vi "Topo & GridSpectr_DriftCorrection_v5 - Cloud.vi"(6 "Internal use":string, 7 "Grid param":T2 {"height (m)" format="%#_6p"; "width (m)" format="%#_6p"; "center Y (m)" format="%#_6p"; "center X (m)" format="%#_6p"}, 8 "Error in (no error)":errorcluster, 9 "Points Y/Index Y":i32, 10 "Points X/Index X":i32, 11 "Method":enum16{"init", "run", "end"}(ring)=enum."end") -> (0 "Error out":errorcluster)   [LabVIEW 2014]
doc: "Example of a measurement VI to be used in the \"Experiments on a Grid\" tool as external VI.\n\nThis example measure the topography and spectroscopy data. The spectroscopy measurements are taken on a subgrid. The data are saved to a sxm and a binary file.\n\n- Nanonis Programming Interface -"
uses:
  <userlib>/Nanonis Prog Interface V5/Nanonis Prog Interface.lvlib
panel:
  in  "Drift Correction":bool
  in  "Set Session":bool
  in  "STS current step":dbl format="%#_6p"
  in  "tip Speed (m/s)":sgl=1e-08 format="%.2p"
  in  "Drift Correction 2":T1
  out "X drift":i32
  out "Y drift":i32
  out "Queue Steps":i32=40
  in  "StepsBack":i32=40
  in  "Channel index (0-23)":u8=14
  in  "File name":string="_3_mol_Chain_single_mol_KONDO"
  in  "STS Current":dbl=2e-10 format="%#_6p"
  in  "Imaging Current":dbl=8e-11 format="%#_6p"
  in  "zdrift \nDuration (s)":dbl
  in  "Correct z drift":bool
  out "Status":string="init"
  in  "Drift correction Pixels":i32=256 caption="Pixels for drift correction"
  out "Y Offset":dbl
  out "X Offset":dbl
  out "Points taken":dbl
  in  "Drift Correction every":i32=10
  in  "Y subgrid spacing":u16=1
  in  "X subgrid spacing":u16=1
  # "drift corr. broken"
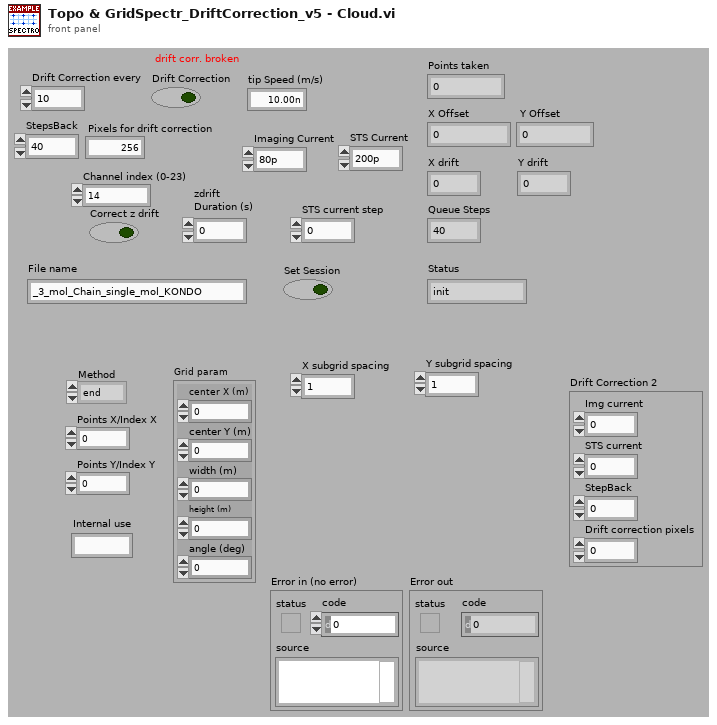
[diagram p1: front panel]
types:
  T1 = cluster{"Img current":dbl, "STS current":dbl, "StepBack":dbl, "Drift correction pixels":dbl}
  T2 = cluster{"center X (m)":sgl, "center Y (m)":sgl, "width (m)":sgl, "height (m)":sgl, "angle (deg)":sgl}
  T3 = enum16{"Header", "TOPO", "STS", "GRID", "GRIDCloud"}
  T4 = cluster{"center X":sgl, "center Y":sgl, "angle":sgl, "width":sgl, "height":sgl, "# pixels":i32, "# lines":i32}
  T5 = cluster{"Name":string, "Calibration":sgl, "Offset":sgl, "Channel index":i32}[]
  T6 = cluster{"up/down":bool, "time/line":sgl, "start time":timestamp, "end time":timestamp}
  T7 = cluster{"Z averaging time (s)":sgl, "Z offset (m)":sgl, "Initial settling time (s)":sgl}
  T8 = cluster{"Max. slew rate (V/s)":sgl, "Settling time (s)":sgl, "Integration time (s)":sgl}
  T9 = cluster{"End settling time (s)":sgl, "Z control time (s)":sgl}
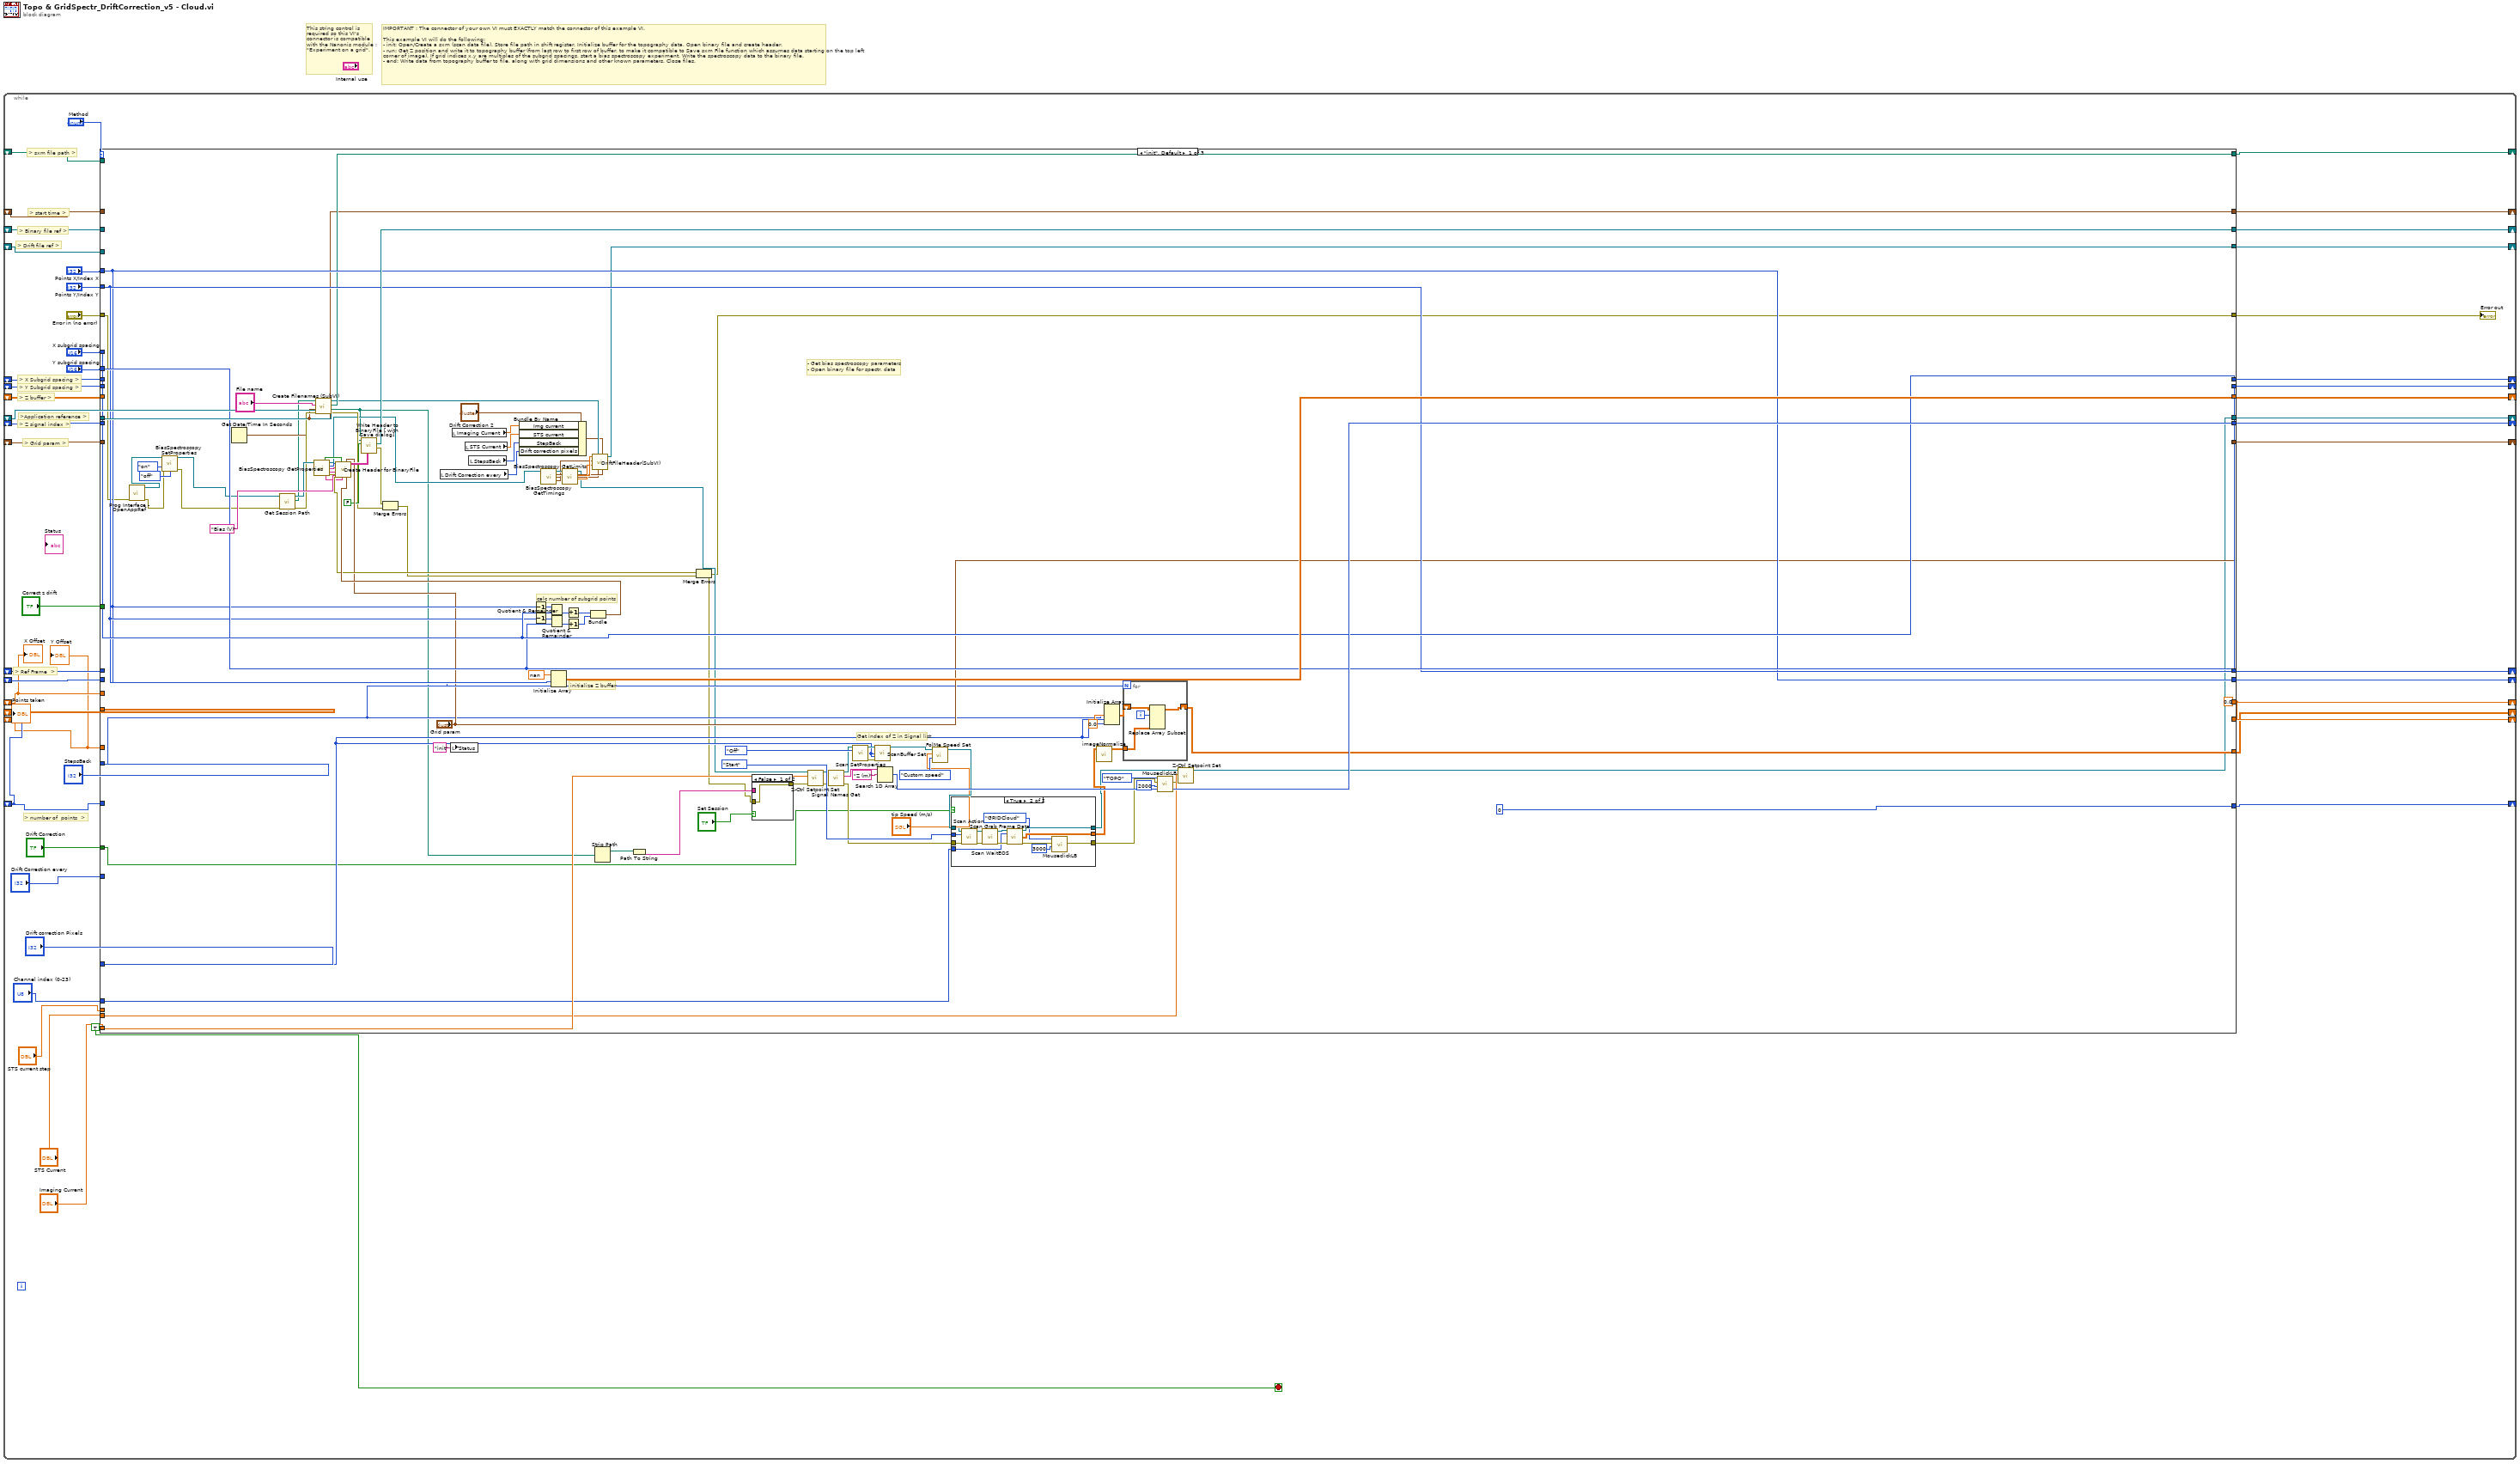
[diagram p0: block diagram]
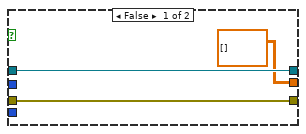
[diagram p2: hidden frame]
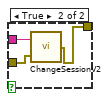
[diagram p3: hidden frame]
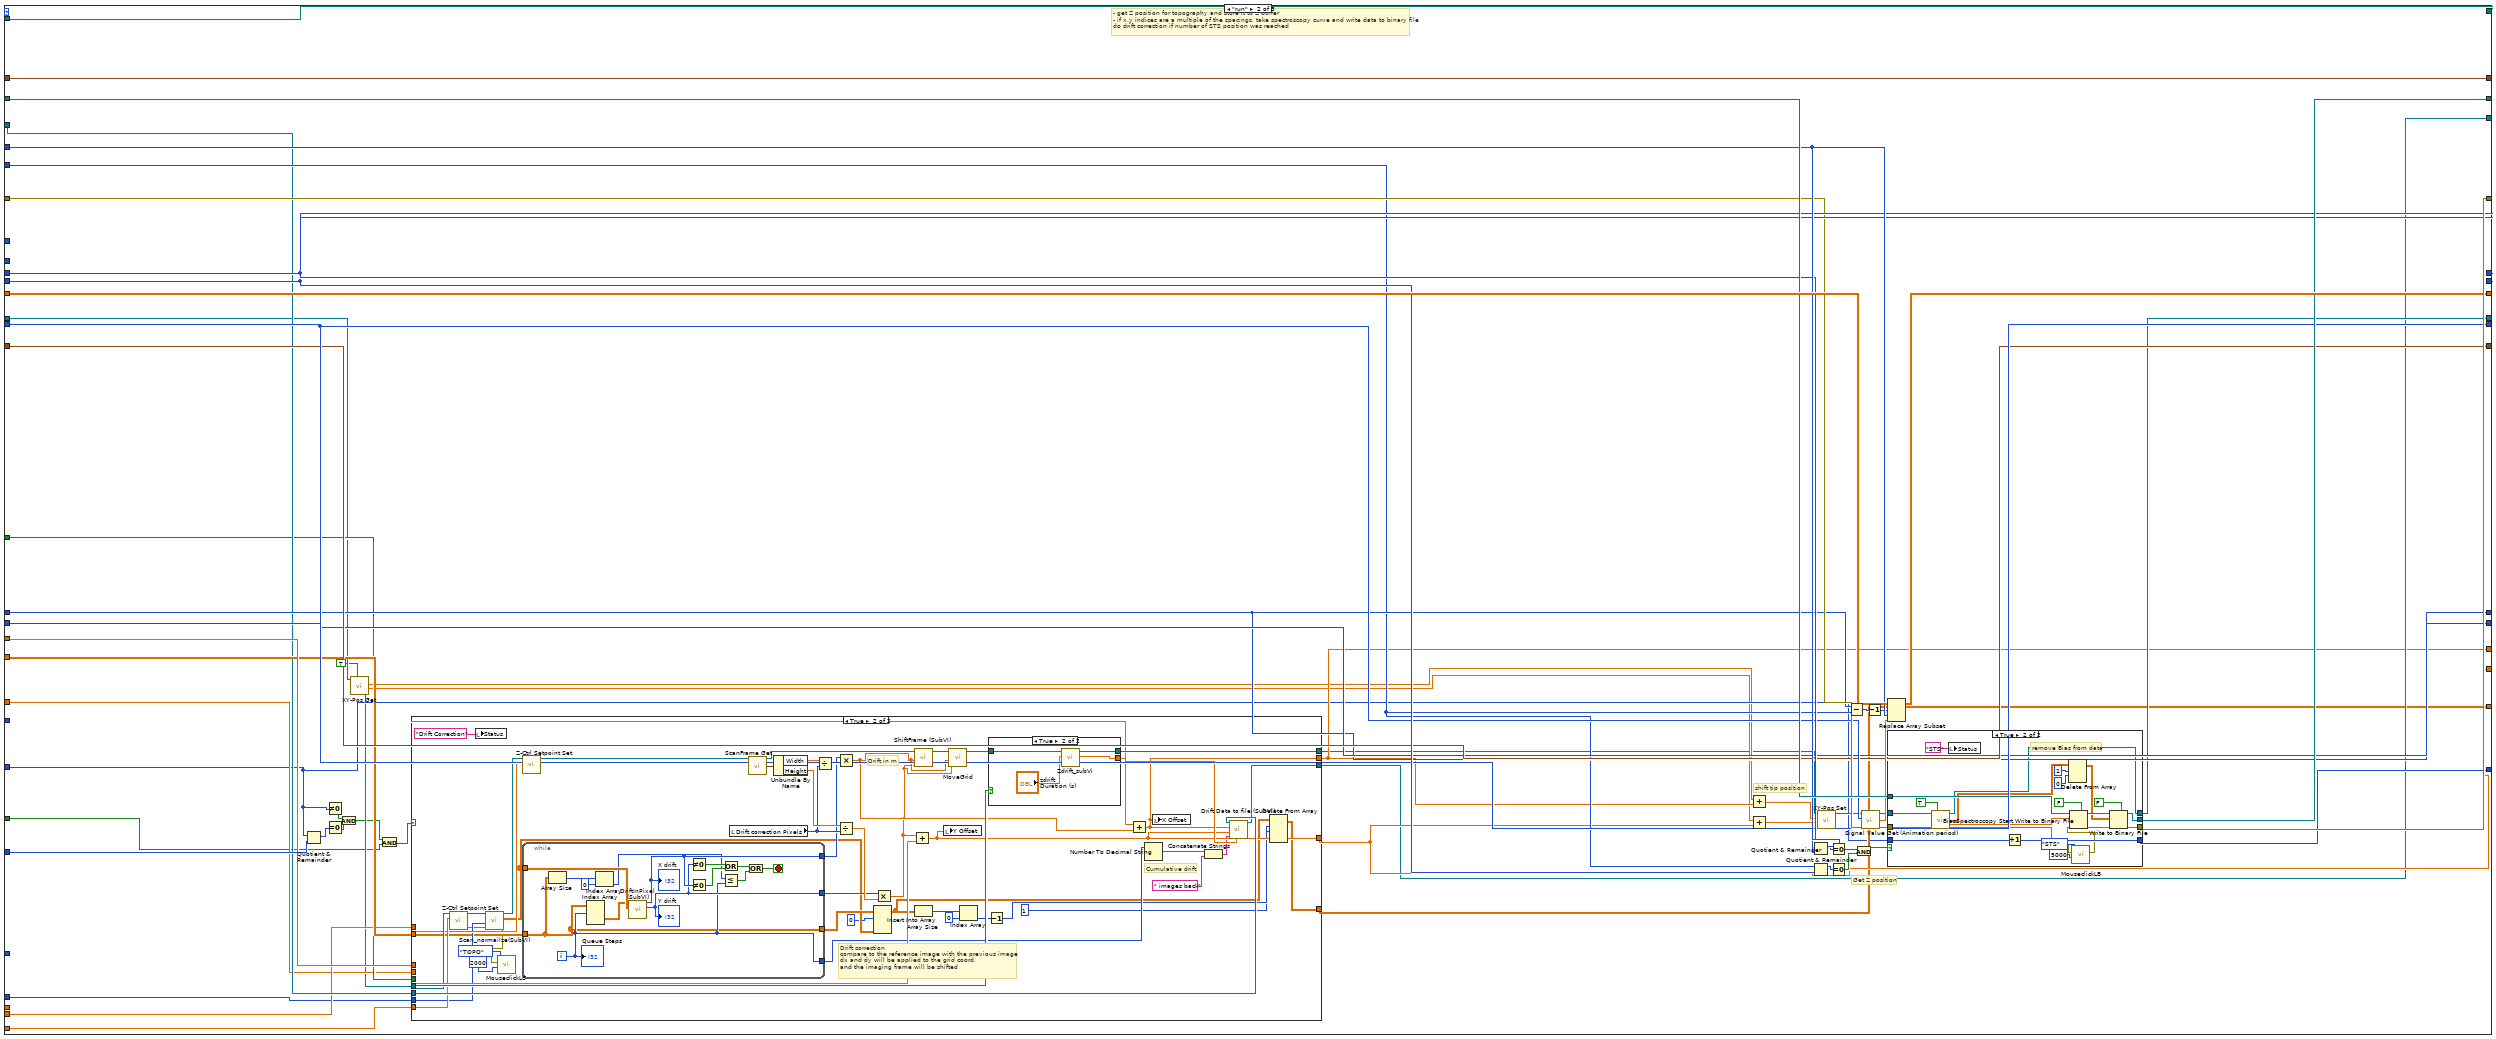
[diagram p4: hidden frame]
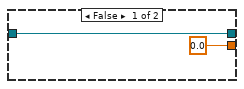
[diagram p6: hidden frame]
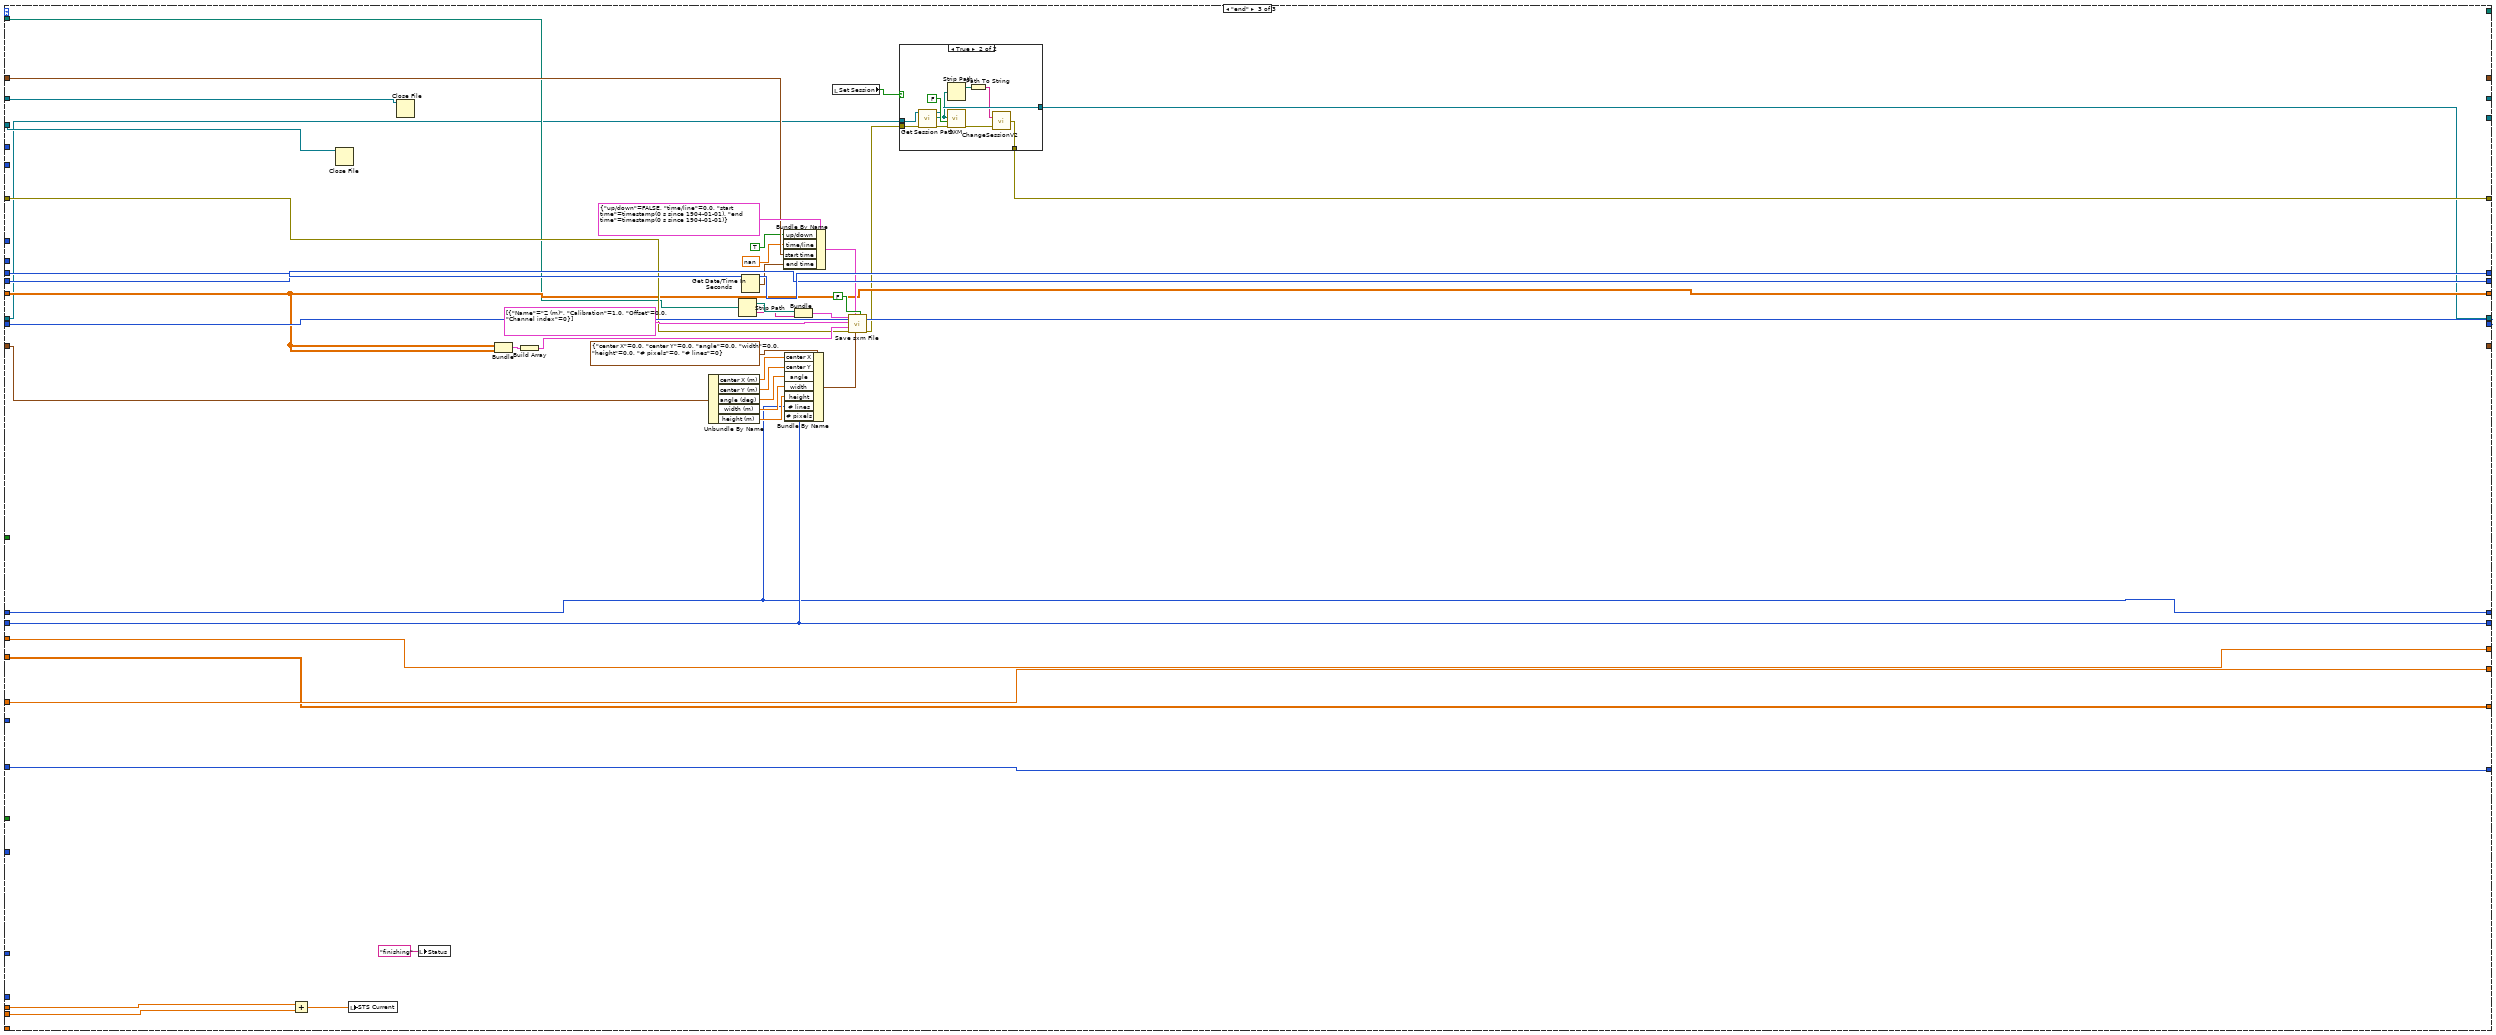
[diagram p8: hidden frame]
diagram:
  # "This string control is required so this VI's connector is compatible with the Nanonis module : \"Experiment on a grid\"."
  # "IMPORTANT : The connector of your own VI must EXACTLY match the connector of this example VI.\n\nThis example VI will do the following:\n- init: Open/Create a sxm (scan data file). Store file path in shift register. Initialize buffer for the topography data. Open binary file and create header.\n- run: Get Z position and write it to topography buffer (from last row to first row of buffer, to make it compatible to Save sxm File function which assumes data starting on the top left corner of image). If grid indices x,y are multiples of the subgrid spacings, start a bias spectroscopy experiment. Write the spectroscopy data to the binary file.\n- end: Write data from topography buffer to file, along with grid dimensions and other known parameters. Close files."
  n1 = while {
    shift-right: [w24] -> _
    shift-left: _ -> [w47]
    shift-right: [w42] -> _
    shift-left: _ -> [w41]
    shift-right: [w39] -> _
    shift-left: _ -> [w40]
    shift-right: [w38] -> _
    shift-left: _ -> [w37]
    shift-right: [w31] -> _
    shift-left: _ -> [w33]
    shift-right: [w32] -> _
    shift-left: _ -> [w34]
    shift-right: [w30] -> _
    shift-left: _ -> [w29]
    shift-right: [w28] -> _
    shift-left: _ -> [w27]
    shift-right: [w26] -> _
    shift-left: _ -> [w25]
    shift-right: [w23] -> _
    shift-left: _ -> [w22]
    shift-right: [w21] -> _
    shift-left: _ -> [w20]
    shift-right: [w19] -> _
    shift-left: _ -> [w12]
    shift-right: [w18] -> _
    shift-left: _ -> [w11]
    shift-right: [w17] -> _
    shift-left: _ -> [w14]
    shift-right: [w16] -> _
    shift-left: _ -> [w13]
    shift-right: [w9] -> _
    shift-left: _ -> [w8]
    stop <- TRUE stop-if-true
    # "> Drift file ref >"
    # "> number of  points  >"
    # "> Ref Frame  >"
    # "> Grid param >"
    # "> start time >"
    # ">Application reference >"
    # "> Y Subgrid spacing >"
    # "> X Subgrid spacing >"
    # "> Z signal index >"
    # "> Binary file ref >"
    # "> Z buffer >"
    # "> sxm file path >"
    n2 = case shown="\"init\", Default" "Method" {
      tunnel: [w102 w228 _] -> w24
      tunnel: w47 -> [_ w228 w336]
      tunnel: "Error in (no error)" -> [w63 w214 w359]
      tunnel: [w57 w227 w333] -> w45
      tunnel: "Points X/Index X" -> [w122 w222 _]
      tunnel: "Points Y/Index Y" -> [w123 w206 _]
      tunnel: [w146 w225 w348] -> w42
      tunnel: w41 -> [_ w226 w348]
      tunnel: w40 -> [_ w224 w337]
      tunnel: [w138 w223 _] -> w39
      tunnel: [w136 w212 w373] -> w38
      tunnel: w37 -> [_ w212 w373]
      tunnel: "X subgrid spacing" -> [w135 _ _]
      tunnel: "Y subgrid spacing" -> [w134 _ _]
      tunnel: w34 -> [_ w216 w372]
      tunnel: w33 -> [_ w215 w371]
      tunnel: [w135 w216 w372] -> w32
      tunnel: [w134 w215 w371] -> w31
      tunnel: [w75 w198 w331] -> w30
      tunnel: w29 -> [_ w180 w332]
      tunnel: ["Grid param" w209 _] -> w28
      tunnel: w27 -> [_ w209 w358]
      tunnel: [w101 w210 _] -> w26
      tunnel: w25 -> [_ w210 w366]
      tunnel: [w123 w207 w349] -> w23
      tunnel: w22 -> [_ w207 w349]
      tunnel: [w122 w208 w350] -> w21
      tunnel: w20 -> [_ w208 w350]
      tunnel: [w117 w188 w347] -> w19
      tunnel: [w117 w193 w345] -> w18
      tunnel: [w96 w185 w341] -> w17
      tunnel: [0 w203 w346] -> w16
      tunnel: w13 -> [_ w182 w346]
      tunnel: "Drift Correction every" -> [_ w201 _]
      tunnel: w14 -> [_ w192 w341]
      tunnel: w12 -> [_ w199 w347]
      tunnel: w11 -> [_ w183 w345]
      tunnel: "Drift correction Pixels" -> [w95 _ _]
      tunnel: [w91 w190 _] -> w9
      tunnel: w8 -> [_ w191 w342]
      tunnel: "Correct z drift" -> [_ w189 _]
      tunnel: "Imaging Current" -> [w108 w187 _]
      tunnel: "STS Current" -> [w105 w186 w338]
      tunnel: "Channel index (0-23)" -> [w99 w184 _]
      tunnel: "StepsBack" -> [w94 _ _]
      tunnel: "STS current step" -> [_ _ w340]
      tunnel: "Drift Correction" -> [w52 w172 _]
      frame "init", Default {
        w117 = 0.0
        # "- Get bias spectroscopy parameters\n- Open binary file for spectr. data"
        # "initialize Z buffer"
        # "calc number of subgrid points"
        # "Get index of Z in Signal list"
        n3 = call <userlib>:"Prog Interface - OpenAppRef.vi"("Error in (no error)"=w63) -> ("Error out"=w62:errorcluster, "Application reference"=w65:refnum<vi>)  [unwired: 5 in]
        n4 = call <userlib>:"BiasSpectroscopy SetProperties.vi"("Application ref in"=w65, "Autosave (no change)"=enum16{"no change", "on", "off"}."on", "Error in (no error)"=w62, "Save dialog"=enum16{"no change", "on", "off"}."off") -> ("Application ref out"=w64:refnum<vi>, "Error out"=w61:errorcluster)  [unwired: 10 in]
        n5 = Get Date/Time In Seconds() -> (seconds since 1Jan1904=w101:timestamp)
        n6 = call <userlib>:"Get Session Path.vi"("error in (no error)"=w61, "Application ref in"=w64) -> ("error out"=w103:errorcluster, "Session path"=w68:path, "Application ref out"=w104:refnum<vi>)  [unwired: 7 in]
        n7 = call <userlib>:"BiasSpectroscopy GetProperties.vi"("Application ref in"=w104) -> ("Backward sweep"=w142:bool, "Application ref out"=w74:refnum<vi>, "Number of points"=w125:i32, "Channels"=w124:string[], "Parameters"=w140:string[], "Fixed parameters"=w127:string[], "Error out"=w139:errorcluster)  [unwired: 6 in, 2 out]
        n8 = call "Create Filenames (SubVI).vi"("error in (no error)"=w103, "seconds since 1Jan1904"=w101, "File name"="File name", "Session path"=w68) -> ("error out"=w76:errorcluster, "binFilePath"=w58:path, "topoFilePath"=w102:path, "Drift File out"=w92:refnum<file>)  [unwired: 4 in]
        n9 = local read "Drift Correction every"() -> (w86:i32)
        n10 = local write "Status"("init" ("Status")) -> ()
        n11 = local read "Imaging Current"() -> (w88:dbl)
        n12 = local read "STS Current"() -> (w87:dbl)
        n13 = local read "StepsBack"() -> (w85:i32)
        n14 = Bundle By Name(cluster="Drift Correction 2", "Img current"=w88, "STS current"=w87, "StepBack"=w85, "Drift correction pixels"=w86) -> (w89:T1)
        n15 = Decrement(x=w122) -> (x-1=w133:i32)
        n16 = Decrement(x=w123) -> (x-1=w132:i32)
        n17 = call <userlib>:"BiasSpectroscopy GetTimings.vi"("Application ref in"=w74) -> ("Application ref out"=w84:refnum<vi>, "Initialization"=w81:T7, "Sweep Timing"=w79:T8, "End of Sweep"=w80:T9)  [unwired: 10 in, 1 out]
        n18 = Quotient & Remainder(x=w133, y=w135) -> (floor(x/y)=w131:i32)  [unwired: 1 out]
        n19 = Quotient & Remainder(x=w132, y=w134) -> (floor(x/y)=w130:i32)  [unwired: 1 out]
        n20 = Initialize Array(sgl nan ("element"), w123, w122) -> (w146:sgl[][])
        n21 = call <userlib>:"BiasSpectroscopy GetLimits.vi"("Application ref in"=w84) -> ("End value (V)"=w82:sgl, "Start value (V)"=w83:sgl, "Application ref out"=w73:refnum<vi>)  [unwired: 5 in, 1 out]
        n22 = Increment(x=w131) -> (x+1=w129:i32)
        n23 = Increment(x=w130) -> (x+1=w128:i32)
        n24 = Bundle(w129, w128) -> (w141:cluster{i32, i32})  [unwired: 1 in]
        n25 = call <userlib>:"Create Header for BinaryFile.vi"("Grid points"=w141, "Grid param"="Grid param", "Fixed parameters"=w127, "Backward sweep"=w142, "Sweep signal"="Bias (V)" ("Sweep Signal"), "Parameters"=w140, "Channels"=w124, "Points per sweep"=w125) -> ("Header (fixed attributes)"=w144:string[][])  [unwired: 3 in]
        n26 = call <userlib>:"Write Header to BinaryFile [ with Save dialog].vi"("Fixed Attributes"=w144, "Show Dialog? (T)"=FALSE, "Filename"=w58) -> ("Error out"=w77:errorcluster, "File ref"=w138:refnum<file>)  [unwired: 5 in, 2 out]
        n27 = Merge Errors(w77, w76) -> (w78:errorcluster)
        n28 = call "DriftFileHeader(SubVI).vi"("Initialization"=w81, "Drift Correction"=w89, "Sweep Timing"=w79, "Byte Stream File in"=w92, "End value (V)"=w82, "End of Sweep"=w80, "Start value (V)"=w83) -> ("Byte Stream File out"=w91:refnum<file>)  [unwired: 4 in]
        n29 = Strip Path(path=w58) -> (stripped path=w60:path)  [unwired: 1 out]
        n30 = Path To String(path=w60) -> (string=w59:string)
        n31 = Merge Errors(w139, w78) -> (w57:errorcluster)
        n32 = case shown="False" "Set Session" {
          tunnel: w59 -> [_ w167]
          tunnel: w57 -> [w164 w166]
          tunnel: [w164 w165] -> w56
          frame False {
          }
          frame True {
            n33 = call "ChangeSessionV2.vi"("error in (no error)"=w166, "Session"=w167) -> ("error out"=w165:errorcluster)
          }
        }
        n34 = call <userlib>:"Z-Ctrl Setpoint Set.vi"("error in (no error)"=w56, "Z Controller setpoint"=w108, "Application ref in"=w73) -> ("error out"=w107:errorcluster, "Application ref out"=w109:refnum<vi>)  [unwired: 7 in]
        n35 = call <userlib>:"Signal Names Get.vi"("error in (no error)"=w107, "Application ref in"=w109) -> ("error out"=w118:errorcluster, "Signals Names"=w126:string[], "Application ref out"=w113:refnum<vi>)  [unwired: 5 in]
        n36 = call <userlib>:"Scan SetProperties.vi"("Application ref in"=w113, "Continuous scan"=enum16{"No change", "On", "Off"}."Off") -> ("Application ref out"=w115:refnum<vi>, "Error out"=w114:errorcluster)  [unwired: 12 in]
        n37 = call <userlib>:"ScanBuffer Set.vi"("Application ref in"=w115, "Pixels"=w95, "Lines"=w95, "error in (no error)"=w114) -> ("Application ref out"=w72:refnum<vi>)  [unwired: 10 in, 1 out]
        n38 = Search 1D Array(1D array=w126, element="Z (m)") -> (index of element=w136:i32)  [unwired: 1 in]
        n39 = call <userlib>:"FolMe Speed Set.vi"("Speed Setting (Custom)"=enum32{"Scan speed", "Custom speed"}."Custom speed", "Speed (m/s)"="tip Speed (m/s)", "Application ref in"=w72) -> ("Application ref out"=w71:refnum<vi>)  [unwired: 5 in, 1 out]
        n40 = case shown="True" w52 {
          tunnel: enum16{"Start", "Stop", "Pause", "Resume"}."Start" ("Scan action (Start)") -> [_ w159]
          tunnel: w118 -> [w149 w158]
          tunnel: [sgl[][] [] ("Scan frame data") w157] -> w110
          tunnel: [w148 w156] -> w106
          tunnel: w99 -> [_ w155]
          tunnel: w71 -> [w148 w154]
          tunnel: [w149 w152] -> w54
          frame False {
          }
          frame True {
            n41 = call <userlib>:"Scan Action.vi"("error in (no error)"=w158, "Scan action (Start)"=w159, "Application ref in"=w154) -> ("error out"=w163:errorcluster, "Application ref out"=w162:refnum<vi>)  [unwired: 6 in]
            n42 = call <userlib>:"Scan WaitEOS.vi"("error in (no error)"=w163, "Application ref in"=w162) -> ("error out"=w160:errorcluster, "Application ref out"=w161:refnum<vi>)  [unwired: 5 in, 2 out]
            n43 = call <userlib>:"Scan Grab Frame Data.vi"("Application ref in"=w161, "Channel index (0-23)"=w155, "error in (no error)"=w160) -> ("Application ref out"=w156:refnum<vi>, "Scan frame data"=w157:sgl[][], "error out"=w153:errorcluster)  [unwired: 8 in, 2 out]
            n44 = call "MouseclickLB.vi"("nMilliseconds"=3000, "error in (no error)"=w153, "Click"=T3."GRIDCloud") -> ("error out"=w152:errorcluster)  [unwired: 8 in]
          }
        }
        n45 = call "imageNormalize.vi"("Data"=w110) -> ("Array"=w93:dbl[][])  [unwired: 10 in]
        n46 = Initialize Array(0.0 ("element"), w94, w95, w95) -> (w97:dbl[][][])
        n47 = for {
          N: w94 -> [_]
          tunnel: w93 -> [w170]
          shift-right: [w169] -> w96
          shift-left: w97 -> [w171]
          i -> [w168]
          n48 = Replace Array Subset(array=w171, new element=w170, index (dim 0)=w168) -> (w169:dbl[][][])  [unwired: 2 in]
        }
        n49 = call "MouseclickLB.vi"("nMilliseconds"=2000, "error in (no error)"=w54, "Click"=T3."TOPO") -> ("error out"=w55:errorcluster)  [unwired: 8 in]
        n50 = call <userlib>:"Z-Ctrl Setpoint Set.vi"("error in (no error)"=w55, "Z Controller setpoint"=w105, "Application ref in"=w106) -> ("Application ref out"=w75:refnum<vi>)  [unwired: 7 in, 1 out]
      }
      frame "run" {
        # "shift tip position"
        # "Get Z position"
        # "- get Z position for topography and store it to Z buffer\n- if x,y indices are a multiple of the spacings, take spectroscopy curve and write data to binary file\ndo drift correction if number of STS position was reached"
        n51 = Quotient & Remainder(x=w182, y=w201) -> (x-y*floor(x/y)=w202:i32)  [unwired: 1 out]
        n52 = Not Equal To 0?(x=w182) -> (x != 0?=w181:bool)
        n53 = Equal To 0?(x=w202) -> (x = 0?=w200:bool)
        n54 = And(x=w181, y=w200) -> (x .and. y?=w174:bool)
        n55 = call <userlib>:"XY-Pos Get.vi"("Wait for newest data (F=False)"=TRUE, "Application ref in"=w180) -> ("Y (m)"=w176:sgl, "X (m)"=w177:sgl, "Application ref out"=w179:refnum<vi>)  [unwired: 5 in, 1 out]
        n56 = And(x=w174, y=w172) -> (x .and. y?=w173:bool)
        n57 = case shown="True" w173 {
          tunnel: w179 -> [w233 w267]
          tunnel: [w233 w273] -> w175
          tunnel: w192 -> [w230 w256]
          tunnel: [w232 w269] -> w188
          tunnel: [w231 w268] -> w193
          tunnel: w199 -> [w232 w271]
          tunnel: w183 -> [w231 w272]
          tunnel: [w230 w248] -> w185
          tunnel: w191 -> [w229 w276]
          tunnel: [w229 w275] -> w190
          tunnel: w189 -> [_ w270]
          tunnel: w187 -> [_ w266]
          tunnel: w186 -> [_ w264]
          tunnel: w184 -> [_ w259]
          frame False {
          }
          frame True {
            # "Cumulative drift"
            # "Drift in m"
            # "Drift correction \ncompare to the reference image with the previous image \ndx and dy will be applied to the grid coord, \nand the imaging frame will be shifted"
            n58 = call <userlib>:"Z-Ctrl Setpoint Set.vi"("Z Controller setpoint"=w266, "Application ref in"=w267) -> ("error out"=w237:errorcluster, "Application ref out"=w263:refnum<vi>)  [unwired: 8 in]
            n59 = local write "Status"("Drift Correction" ("Status")) -> ()
            n60 = call "Scan_normailze(SubVI).vi"("error in (no error)"=w237, "Channel index (0-23)"=w259, "Application in"=w263) -> ("error out"=w236:errorcluster, "Array"=w250:dbl[][], "Application out"=w265:refnum<vi>)  [unwired: 6 in]
            n61 = call "MouseclickLB.vi"("nMilliseconds"=2000, "error in (no error)"=w236, "Click"=enum16{"Header", "TOPO", "STS", "GRID"}."TOPO") -> ()  [unwired: 8 in, 1 out]
            n62 = call <userlib>:"Z-Ctrl Setpoint Set.vi"("Z Controller setpoint"=w264, "Application ref in"=w265) -> ("Application ref out"=w261:refnum<vi>)  [unwired: 8 in, 1 out]
            n63 = while {
              tunnel: w250 -> [w294]
              tunnel: w256 -> [w284]
              tunnel: [w293] -> w258
              tunnel: [w292] -> w257
              tunnel: [w288] -> w255
              tunnel: [w284] -> w251
              i -> [w288]
              stop <- w290 stop-if-true
              n64 = Array Size(array=w284) -> (size(s)=w287:i32[])
              n65 = Index Array(array=w284, index (dim 0)=w288) -> (element=w283:dbl[][])  [unwired: 2 in]
              n66 = Index Array(array=w287, index=0) -> (element=w285:i32)
              n67 = call "DriftInPixel (SubVI).vi"("New image"=w294, "Ref image"=w283) -> ("Y drift"=w292:i32, "X drift"=w293:i32)  [unwired: 7 in, 1 out]
              "Y drift" <- w292
              "X drift" <- w293
              n68 = Not Equal To 0?(x=w292) -> (x != 0?=w296:bool)
              n69 = Not Equal To 0?(x=w293) -> (x != 0?=w295:bool)
              n70 = Or(x=w296, y=w295) -> (x .or. y?=w291:bool)
              n71 = Less Or Equal?(x=w285, y=w288) -> (x <= y?=w289:bool)
              n72 = Or(x=w291, y=w289) -> (x .or. y?=w290:bool)
              "Queue Steps" <- w288
            }
            n73 = local read "Drift correction Pixels"() -> (w260:i32)
            n74 = call <userlib>:"ScanFrame Get.vi"("Application ref in"=w261) -> ("Application ref out"=w262:refnum<vi>, "Size (m)"=w281:cluster{"Width":sgl, "Height":sgl})  [unwired: 10 in, 3 out]
            n75 = Unbundle By Name(w281) -> ("Width"=w280:sgl, "Height"=w282:sgl)
            n76 = Divide(x=w280, y=w260) -> (x/y=w279:sgl)
            n77 = Divide(x=w282, y=w260) -> (x/y=w278:sgl)
            n78 = Multiply(x=w258, y=w279) -> (x*y=w239:sgl)
            n79 = Insert Into Array(array=w251, index (dim 0)=0 ("index (page)"), new element=w250) -> (w247:dbl[][][])  [unwired: 2 in]
            n80 = Multiply(x=w257, y=w278) -> (x*y=w238:sgl)
            n81 = Add(x=w238, y=w272) -> (x+y=w268:dbl)
            n82 = call "ShiftFrame (SubVI).vi"("Y shift"=w238, "X shift"=w239, "Application in"=w262) -> ("Application out"=w241:refnum<vi>)  [unwired: 8 in]
            n83 = Array Size(array=w247) -> (size(s)=w246:i32[])
            n84 = local write "Y Offset"(w268) -> ()
            n85 = call "MoveGrid.vi"("y"=w238, "x"=w239, "Application ref in"=w241) -> ("Application ref out"=w240:refnum<vi>)  [unwired: 7 in, 1 out]
            n86 = Index Array(array=w246, index=0) -> (element=w244:i32)
            n87 = Decrement(x=w244) -> (x-1=w243:i32)
            n88 = case shown="True" w270 {
              tunnel: [0.0 ("z drift") w302] -> w274
              tunnel: w240 -> [w297 w301]
              tunnel: [w297 w300] -> w273
              frame False {
              }
              frame True {
                n89 = call "Zdrift_subVi.vi"("Duration"="zdrift \nDuration (s)", "Application in"=w301) -> ("z drift"=w302:dbl, "Application out"=w300:refnum<vi>)  [unwired: 7 in, 1 out]
              }
            }
            n90 = Add(x=w271, y=w239) -> (x+y=w269:dbl)
            n91 = Number To Decimal String(number=w255) -> (decimal integer string=w254:string)  [unwired: 1 in]
            n92 = local write "X Offset"(w269) -> ()
            n93 = Concatenate Strings(w254, " images back" ("string")) -> (w253:string)
            n94 = call "Drift Data to file (SubVI).vi"("z drift"=w274, "Comment"=w253, "y Drift"=w268, "X drift"=w269, "Byte Stream File in"=w276) -> ("Byte Stream File out"=w275:refnum<file>)  [unwired: 6 in]
            n95 = Delete From Array(array=w247, length=1, index (dim 0)=w243) -> (array with subset deleted=w248:dbl[][][])  [unwired: 2 in, 1 out]
          }
        }
        n96 = Add(x=w177, y=w188) -> (x+y=w195:dbl)
        n97 = Add(x=w176, y=w193) -> (x+y=w194:dbl)
        n98 = Quotient & Remainder(x=w222, y=w216) -> (x-y*floor(x/y)=w221:i32)  [unwired: 1 out]
        n99 = Quotient & Remainder(x=w206, y=w215) -> (x-y*floor(x/y)=w220:i32)  [unwired: 1 out]
        n100 = call <userlib>:"XY-Pos Set.vi"("Y (m)"=w194, "X (m)"=w195, "Application ref in"=w175) -> ("Application ref out"=w196:refnum<vi>)  [unwired: 5 in, 1 out]
        n101 = Equal To 0?(x=w221) -> (x = 0?=w219:bool)
        n102 = Equal To 0?(x=w220) -> (x = 0?=w218:bool)
        n103 = Subtract(x=w207, y=w206) -> (x-y=w205:i32)
        n104 = And(x=w219, y=w218) -> (x .and. y?=w217:bool)
        n105 = call <userlib>:"Signal Value Get (Animation period).vi"("error in (no error)"=w214, "Signal index (0-47)"=w212, "Application ref in"=w196) -> ("error out"=w213:errorcluster, "Signal value"=w211:sgl, "Application ref out"=w197:refnum<vi>)  [unwired: 5 in]
        n106 = Decrement(x=w205) -> (x-1=w204:i32)
        n107 = Replace Array Subset(array=w226, new element=w211, index (row)=w204, index (col)=w222) -> (w225:sgl[][])
        n108 = case shown="True" w217 {
          tunnel: [w305 w314] -> w227
          tunnel: w224 -> [w306 w329]
          tunnel: [w306 w327] -> w223
          tunnel: w213 -> [w305 w326]
          tunnel: w197 -> [w304 w318]
          tunnel: [w304 w317] -> w198
          tunnel: [w303 w312] -> w203
          tunnel: w182 -> [w303 w313]
          frame False {
            # "Point indices aren't multiple of subgrid spacing\n=> no spectroscopy at this point"
          }
          frame True {
            # "remove Bias from data"
            n109 = call <userlib>:"BiasSpectroscopy Start.vi"("Application ref in"=w318, "Get data (F)"=TRUE ("Get Data (F)"), "Error in (no error)"=w326) -> ("Application ref out"=w317:refnum<vi>, "Data"=w325:sgl[][], "Parameters"=w324:sgl[], "Error out"=w309:errorcluster)  [unwired: 8 in, 1 out]
            n110 = local write "Status"("STS" ("Status")) -> ()
            n111 = Increment(x=w313) -> (x+1=w312:i32)
            n112 = Delete From Array(array=w325, length=1, index (row)=0 ("index")) -> (array with subset deleted=w323:sgl[][])  [unwired: 1 in, 1 out]
            n113 = call "MouseclickLB.vi"("nMilliseconds"=5000, "error in (no error)"=w309, "Click"=enum16{"Header", "TOPO", "STS", "GRID"}."STS") -> ("error out"=w310:errorcluster)  [unwired: 8 in]
            n114 = Write to Binary File(file (use dialog)=w329, data=w324, error in=w310, 5:FALSE ("prepend array or string size? (T)")) -> (refnum out=w328:refnum<file>, error out=w315:errorcluster)  [unwired: 2 in, 1 out]
            n115 = Write to Binary File(file (use dialog)=w328, data=w323, error in=w315, 5:FALSE ("prepend array or string size? (T)")) -> (refnum out=w327:refnum<file>, error out=w314:errorcluster)  [unwired: 2 in, 1 out]
          }
        }
      }
      frame "end" {
        n116 = Add(x=w340, y=w338) -> (x+y=w339:dbl)
        n117 = Close File(refnum=w342) -> ()  [unwired: 1 in, 2 out]
        n118 = local write "STS Current"(w339) -> ()
        n119 = Close File(refnum=w337) -> ()  [unwired: 1 in, 2 out]
        n120 = local write "Status"("finishing" ("Status")) -> ()
        n121 = Bundle(w348, w348) -> (w370:cluster{sgl[][], sgl[][]})  [unwired: 1 in]
        n122 = Build Array(w370) -> (w369:cluster{sgl[][], sgl[][]}[])
        n123 = Unbundle By Name(w358) -> ("center X (m)"=w356:sgl, "center Y (m)"=w355:sgl, "angle (deg)"=w354:sgl, "width (m)"=w353:sgl, "height (m)"=w352:sgl)
        n124 = Strip Path(path=w336) -> (stripped path=w362:path, name=w361:string)
        n125 = Get Date/Time In Seconds() -> (seconds since 1Jan1904=w344:timestamp)
        n126 = Bundle By Name(cluster=T6 {"up/down"=FALSE, "time/line"=0.0, "start time"=timestamp(0 s since 1904-01-01), "end time"=timestamp(0 s since 1904-01-01)} ("Scan param"), "up/down"=TRUE, "time/line"=sgl nan ("input 7"), "start time"=w366, "end time"=w344) -> (w365:T6)
        n127 = Bundle By Name(cluster=T4 {"center X"=0.0, "center Y"=0.0, "angle"=0.0, "width"=0.0, "height"=0.0, "# pixels"=0, "# lines"=0} ("Scanfield"), "center X"=w356, "center Y"=w355, "angle"=w354, "width"=w353, "height"=w352, "# lines"=w349, "# pixels"=w350) -> (w351:T4)
        n128 = Bundle("stripped path"=w362, "name"=w361) -> (w360:cluster{"stripped path":path, "name":string})  [unwired: 1 in]
        n129 = local read "Set Session"() -> (w330:bool)
        n130 = call <userlib>:"Save sxm File.vi"("Auto file naming? (T)"=FALSE, "Scanfield"=w351, "Scan param"=w365, "error in (no error)"=w359, "Channels data"=w369, "Channels config"=T5 [{"Name"="Z (m)", "Calibration"=1.0, "Offset"=0.0, "Channel index"=0}], "Filename control"=w360) -> ("error out"=w334:errorcluster)  [unwired: 2 in, 2 out]
        n131 = case shown="True" w330 {
          tunnel: w334 -> [w374 w383]
          tunnel: [w374 w382] -> w333
          tunnel: w332 -> [w375 w380]
          tunnel: [w375 w379] -> w331
          frame False {
          }
          frame True {
            n132 = call <userlib>:"Get Session Path.vi"("error in (no error)"=w383, "Application ref in"=w380) -> ("error out"=w385:errorcluster, "Session path"=w378:path, "Application ref out"=w379:refnum<vi>)  [unwired: 7 in]
            n133 = Strip Path(path=w378) -> (stripped path=w377:path)  [unwired: 1 out]
            n134 = call "SXM.vi"("Path"=w378, "Delete"=FALSE, "error in"=w385) -> ("error out"=w384:errorcluster)  [unwired: 7 in]
            n135 = Path To String(path=w377) -> (string=w376:string)
            n136 = call "ChangeSessionV2.vi"("error in (no error)"=w384, "Session"=w376) -> ("error out"=w382:errorcluster)
          }
        }
      }
    }
    "Error out" <- w45
    "Points taken" <- w13
    "X Offset" <- w12
    "Y Offset" <- w11
  }
